vi "Robot Global Data.vi"() -> ()   [LabVIEW 2016]
doc: "This global VI can contain as many global variables as you need. Place a control on the panel, give it a good name. To read or write to it from a VI, drag the icon to the diagram of that VI. You can also drag from the project. Click on the node to change which global you access. You shouldn't have multiple locations writing to a global or it will cause a race-condition."
uses:
  <vilib>/Rock Robotics/WPI/Camera/WPI_CameraImageSize.ctl
  <vilib>/Rock Robotics/WPI/DriverStation/WPI_DriverStationRobotMode2.ctl
panel:
  in  "Intake Speed":dbl=0.8
  in  "Hopper Far":dbl=0.75
  in  "Hopper Close":dbl=0.6
  in  "FF Close Tele":dbl=0.66
  in  "FF Far Tele":dbl=0.7
  in  "FF B40":dbl=0.7
  in  "FF B10 G":dbl=0.72
  in  "FF R60 P1":dbl=0.71
  in  "FF R60 P2":dbl=0.704
  in  "B40yDepth":dbl=62.0
  in  "R60P2yDepth":dbl=-74.0
  in  "R60P1yDepth":dbl=-60.0
  in  "center gear depth":dbl=31.0
  in  "Autoaim fast":dbl=0.25
  in  "Autoaim mid":dbl=0.2
  in  "Autoaim slow":dbl=0.19
  in  "Camera Target":dbl=0.06
  out "gear Depth? left":bool
  out "gearDepthraw left":dbl
  in  "hopper far":dbl=0.75
  out "target dist":dbl
  out "slider":dbl
  in  "feed forward far":dbl=0.725
  out "headingF":dbl
  in  "auto":i32=5
  out "offset heading":dbl
  out "finished aim?":bool
  out "center Y":dbl
  out "center X":dbl
  out "autoaim":bool
  out "ramp down":dbl
  out "GEAR-RETAINER":bool
  out "GEAR-SHOVER":bool
  out "Trim Close":dbl=1.0
  out "Trim Far":dbl=1.0
  in  "Trim Close Raw":dbl(knob) scale=-1.0..1.0
  out "Climb NUM":i32
  in  "Climb 2":bool
  out "Arm NUM":i16=1
  in  "Arm Stow":bool=TRUE
  out "have Gear?":bool
  out "gear Depth? right":bool
  out "gearDepthraw right":dbl
  out "gearSense raw":dbl
  out "encShootSpeed":dbl
  out "encHopSpeed":dbl
  out "encShootPos":dbl=-0.0
  out "encHopPos":dbl
  out "encYpos":dbl=-0.0
  in  "Shot Distance":bool=TRUE
  in  "Trim Far Raw":dbl(knob) scale=-1.0..1.0
  in  "Gear Eject":bool
  in  "Climb":bool
  in  "Arm 2":bool=TRUE
  in  "Arm 1":bool=TRUE
  in  "Shoot!":bool
  in  "Spinup shooter":bool
  in  "Intake":bool
  out "driveMode":i32
  out "halo":bool
  out "encXpos":dbl=-0.0
  out "strafeStraight":bool
  out "fieldcentric":bool
  out "resetgyro":bool
  out "z":dbl
  out "y":dbl=-0.0
  out "x":dbl
  out "heading":dbl
  in  "Robot Mode":T1=enum."Finish"
  in  "image size":T2=enum."320x240"
  in  "Enable Vision":bool
  # "Fudge numbers - read from dash"
  # "0 - normal\n1 - hold heading\n2 - halo auto rotate"
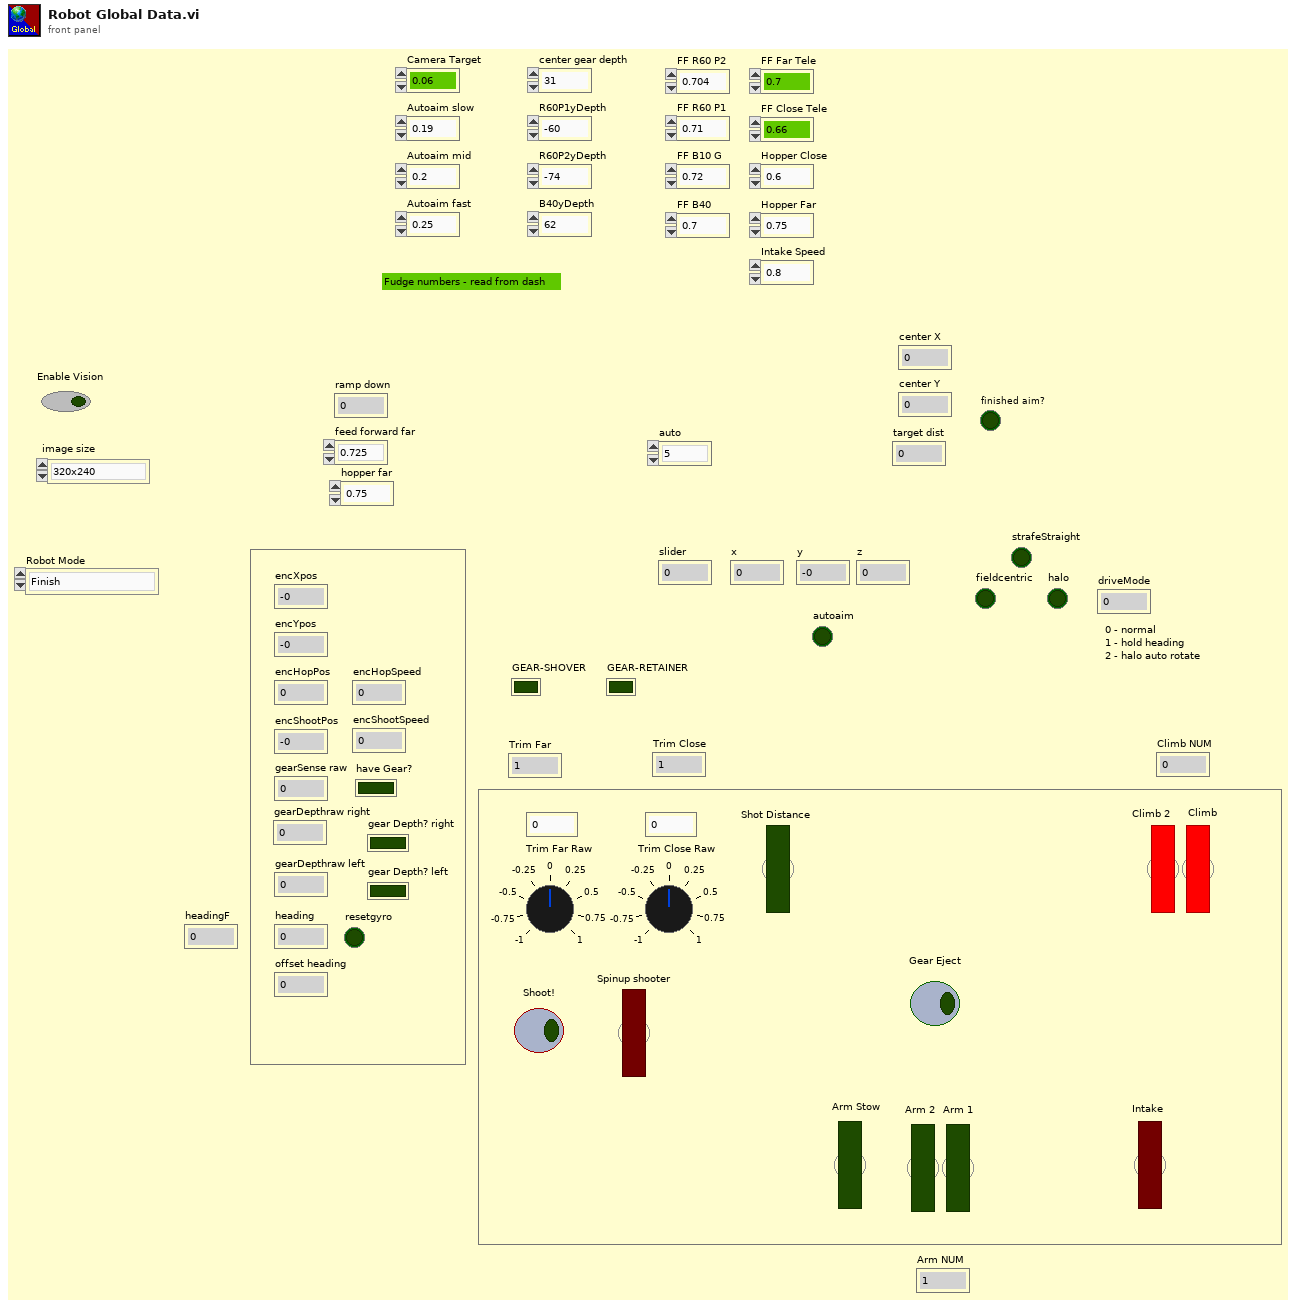
[diagram p1: front panel]
types:
  T1 = typedef "WPI_DriverStationRobotMode2.ctl" = enum16{"Autonomous Disabled", "Autonomous Enabled", "Teleop Disabled", "Teleop Enabled", "Disconnected", "Finish", "Test Disabled", "Test Enabled", "Emergency Stopped"}
  T2 = typedef "WPI_CameraImageSize.ctl" = enum16{"640x480", "320x240", "160x120", "Custom"}
diagram:
